vi "Write alert setting file.vi"(8 "Error In":errorcluster, 10 "Alert setting":T1 {"Temperature High" format="%#.2g°C"; "Humidity High" format="%#.2g%"; "Low battery" min=0.0 max=4.2 step=0.05 format="%#.2gV"; "Temperature Low" format="%#.2g°C"; "Humidity Low" format="%#.2g%"}) -> (0 "Error Out":errorcluster)   [LabVIEW 2016]
uses:
  <vilib>/Utility/config.llb/Write Key (Boolean).vi
  <vilib>/Utility/config.llb/Write Key (Double).vi
  <vilib>/Utility/config.llb/Write Key (String).vi
  <vilib>/Utility/config.llb/NI_LVConfig.lvlib
panel:
  # "Alert Threshold"
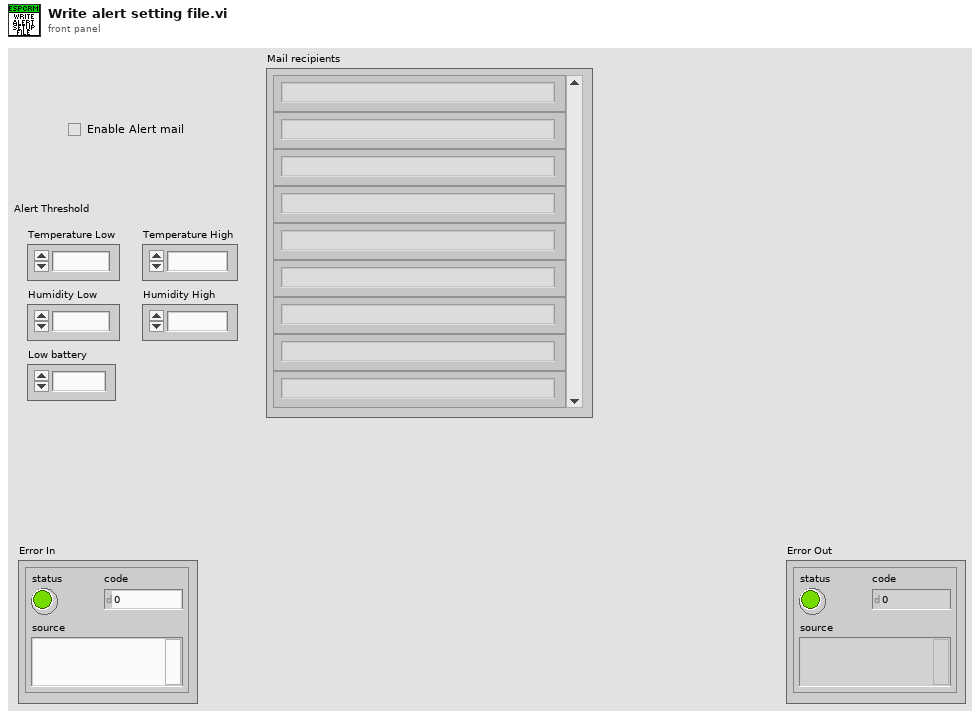
[diagram p1: front panel]
types:
  T1 = cluster{"Mail recipients":string[], "Enable":bool, "Low battery":dbl, "Temperature Low":dbl, "Humidity Low":dbl, "Humidity High":dbl, "Temperature High":dbl}
  T2 = typedef "NI_LVConfig.lvlib/Config Data RefNum.ctl" = refnum<k1>
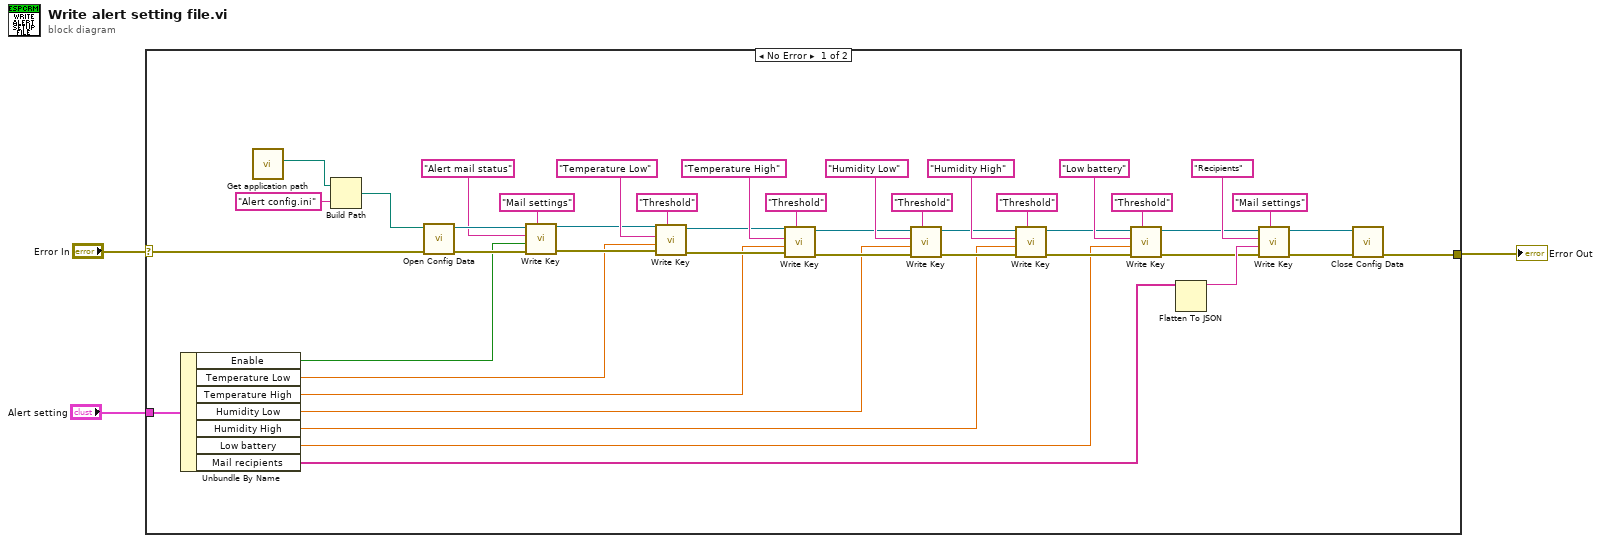
[diagram p0: block diagram]
diagram:
  n1 = case shown="No Error" "Error In" {
    selector: "Error In" -> [w23 w48]
    tunnel: [w22 w48] -> w2
    tunnel: "Alert setting" -> [w11 _]
    frame No Error {
      n2 = Unbundle By Name(w11) -> ("Enable"=w10:bool, "Temperature Low"=w9:dbl, "Temperature High"=w8:dbl, "Humidity Low"=w7:dbl, "Humidity High"=w6:dbl, "Low battery"=w5:dbl, "Mail recipients"=w4:string[])
      n3 = call "Get application path.vi"() -> ("Application path"=w43:path)  [unwired: 11 in]
      n4 = Build Path(base path=w43, name or relative path="Alert config.ini") -> (appended path=w41:path)
      n5 = call <vilib>:"Open Config Data.vi"("error in (no error)"=w23, "configuration file path"=w41) -> ("error out"=w47:errorcluster, "refnum"=w46:T2)  [unwired: 7 in, 1 out]
      n6 = call-poly <vilib>:"Write Key.vi"("section"="Mail settings", "error in (no error)"=w47, "value"=w10, "key"="Alert mail status", "refnum"=w46) -> ("error out"=w31:errorcluster, "refnum out"=w32:T2)  [unwired: 4 in, 1 out]
      n7 = call-poly <vilib>:"Write Key.vi"("section"="Threshold", "error in (no error)"=w31, "value"=w9, "key"="Temperature Low", "refnum"=w32) -> ("error out"=w18:errorcluster, "refnum out"=w19:T2)  [unwired: 4 in, 1 out]
      n8 = call-poly <vilib>:"Write Key.vi"("section"="Threshold", "error in (no error)"=w18, "value"=w8, "key"="Temperature High", "refnum"=w19) -> ("error out"=w14:errorcluster, "refnum out"=w15:T2)  [unwired: 4 in, 1 out]
      n9 = call-poly <vilib>:"Write Key.vi"("section"="Threshold", "error in (no error)"=w14, "value"=w7, "key"="Humidity Low", "refnum"=w15) -> ("error out"=w13:errorcluster, "refnum out"=w12:T2)  [unwired: 4 in, 1 out]
      n10 = call-poly <vilib>:"Write Key.vi"("section"="Threshold", "error in (no error)"=w13, "value"=w6, "key"="Humidity High", "refnum"=w12) -> ("error out"=w24:errorcluster, "refnum out"=w25:T2)  [unwired: 4 in, 1 out]
      n11 = call-poly <vilib>:"Write Key.vi"("section"="Threshold", "error in (no error)"=w24, "value"=w5, "key"="Low battery", "refnum"=w25) -> ("error out"=w27:errorcluster, "refnum out"=w26:T2)  [unwired: 4 in, 1 out]
      n12 = Flatten To JSON(anything=w4) -> (JSON string=w30:string)  [unwired: 2 in, 1 out]
      n13 = call-poly <vilib>:"Write Key.vi"("section"="Mail settings", "error in (no error)"=w27, "value"=w30, "key"="Recipients", "refnum"=w26) -> ("error out"=w34:errorcluster, "refnum out"=w35:T2)  [unwired: 4 in, 1 out]
      n14 = call <vilib>:"Close Config Data.vi"("error in (no error)"=w34, "refnum"=w35) -> ("error out"=w22:errorcluster)  [unwired: 8 in, 1 out]
    }
    frame Error {
    }
  }
  "Error Out" <- w2
